vi "Display and Log Temp.vi"() -> ()   [LabVIEW 2015]
doc: "This VI is used as a subVI in the Temperature System exercise in the LabVIEW Basics I course."
uses:
  <vilib>/Utility/file.llb/Write To Spreadsheet File (DBL).vi
panel:
  in  "Return":bool
  out "Temperature History":dbl(graph)
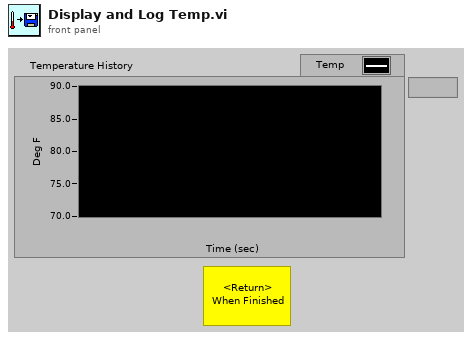
[diagram p1: front panel]
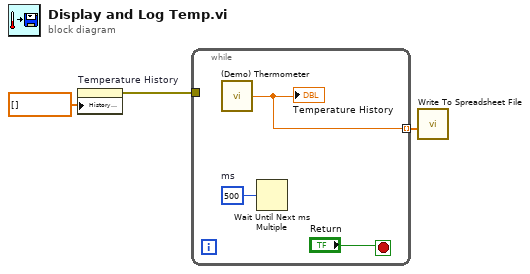
[diagram p0: block diagram]
diagram:
  n1 = property on="Temperature History" class="WFChart (strict)"("History Data"=dbl[] []) -> (error out=w1:errorcluster)  [unwired: 2 in, 1 out]
  n2 = while {
    tunnel: [w5] -> w3 mode=indexing
    tunnel: w1 -> [_]
    stop <- "Return" stop-if-true
    w6 = u32 500  # ms
    n3 = call "(Demo) Thermometer.vi"() -> ("Temperature"=w5:dbl)  [unwired: 1 in]
    "Temperature History" <- w5
    n4 = Wait Until Next ms Multiple(millisecond multiple=w6) -> ()  [unwired: 1 out]
  }
  n5 = call-poly <vilib>:"Write To Spreadsheet File.vi"("1D data"=w3) -> ()  [unwired: 7 in, 1 out]
